vi "geve-msg_serial_config_update.vi"(8 "error in (no error)":errorcluster, 10 "Serial Port Configuration":T1={"timeout (ms)"=0, "VISA resource name"="", "baud rate"=0, "max expected byte count"=128}, 11 "Runtime Data":T2) -> (0 "error out":errorcluster, 3 "Runtime Data out":T2)   [LabVIEW 2018]
doc: "enqueue update serial com action"
uses:
  geve-runtime_data_cluster.ctl
  geve-monitoring_data_cluster.ctl
  geve-serial_config_cluster.ctl
  geve-com_ref_cluster.ctl
  geve-message_cluster.ctl
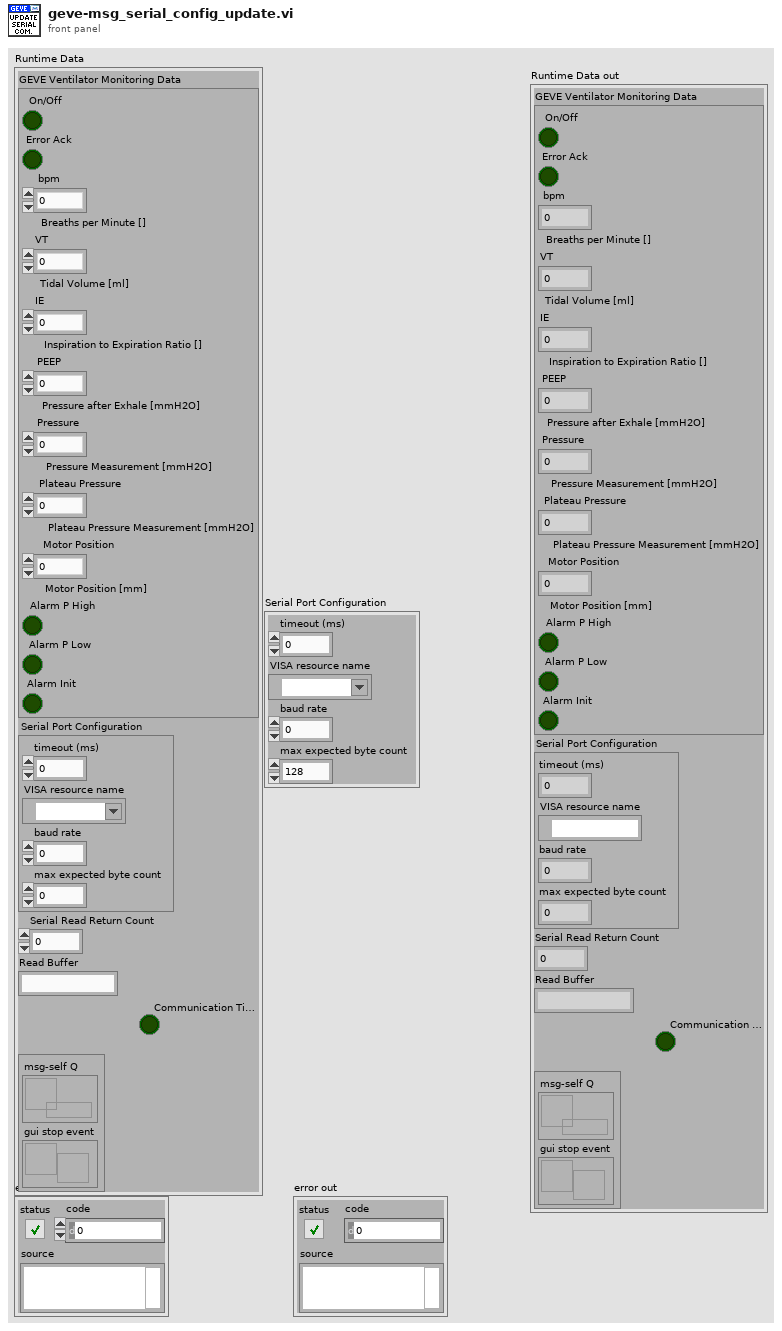
[diagram p1: front panel]
types:
  T1 = typedef "geve-serial_config_cluster.ctl" = cluster{"timeout (ms)":u32, "VISA resource name":refnum<visa-resource-name>, "baud rate":u32, "max expected byte count":u32}
  T2 = typedef "geve-runtime_data_cluster.ctl" = cluster{"GEVE Ventilator Monitoring Data":T3, "Serial Port Configuration":T1, "Serial Read Return Count":u32, "Read Buffer":string, "Communication Timeout?":bool, "com-refs":T4}
  T3 = typedef "geve-monitoring_data_cluster.ctl" = cluster{"On/Off":bool, "Error Ack":bool, "bpm":dbl, "VT":dbl, "IE":dbl, "PEEP":dbl, "Pressure":dbl, "Plateau Pressure":dbl, "Motor Position":dbl, "Alarm P High":bool, "Alarm P Low":bool, "Alarm Init":bool}
  T4 = typedef "geve-com_ref_cluster.ctl" = cluster{"msg-self Q":refnum<queue>, "gui stop event":refnum<user-event>}
  T5 = typedef "geve-message_cluster.ctl" = cluster{"Command":string, "Payload":variant}
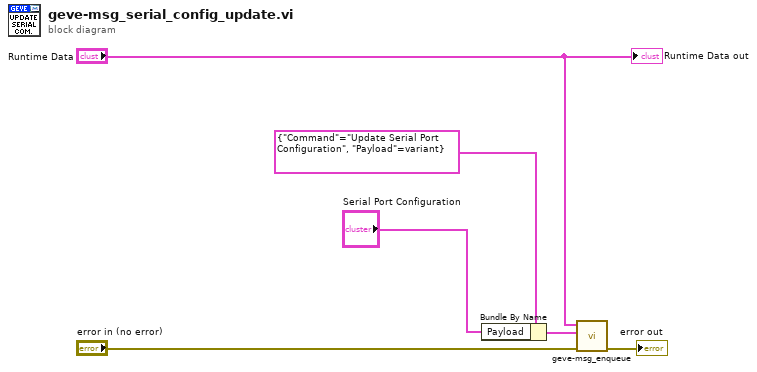
[diagram p0: block diagram]
diagram:
  n1 = Bundle By Name(cluster=T5 {"Command"="Update Serial Port Configuration", "Payload"=variant} ("Message"), "Payload"="Serial Port Configuration") -> (w6:T5)
  n2 = call "geve-msg_enqueue.vi"("error in (no error)"="error in (no error)", "Message"=w6, "Runtime Data"="Runtime Data") -> ("error out"=→"error out":errorcluster)  [unwired: 7 in, 1 out]
  "Runtime Data out" <- "Runtime Data"
